vi "Taller 1 punto 4.vi"() -> ()   [LabVIEW 2017]
panel:
  out "Banda":dbl(slide) scale=0.0..1200.0
  in  "stop":bool
  in  "Velocidad (m/300ms)":dbl(knob) scale=0.0..10.0
  in  "Dirección":bool
  # "TALLER 1, PUNTO 4\nLUZ ANDREA JARAMILLO CASTILLO"
  # "Derecha"
  # "Izquierda"
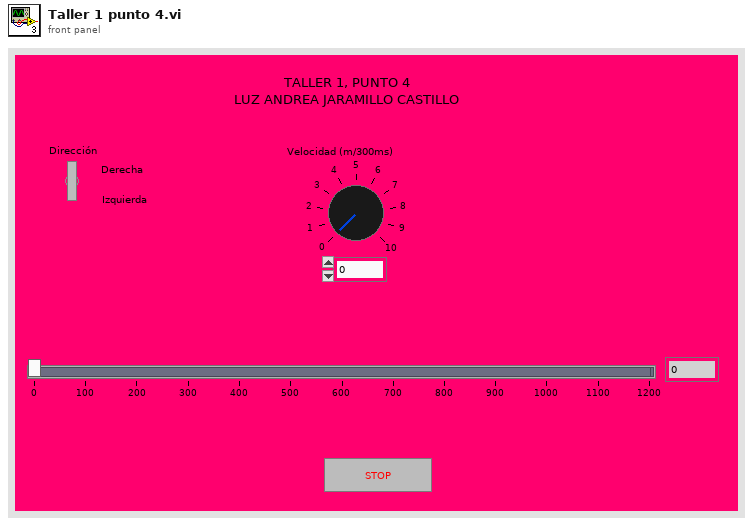
[diagram p1: front panel]
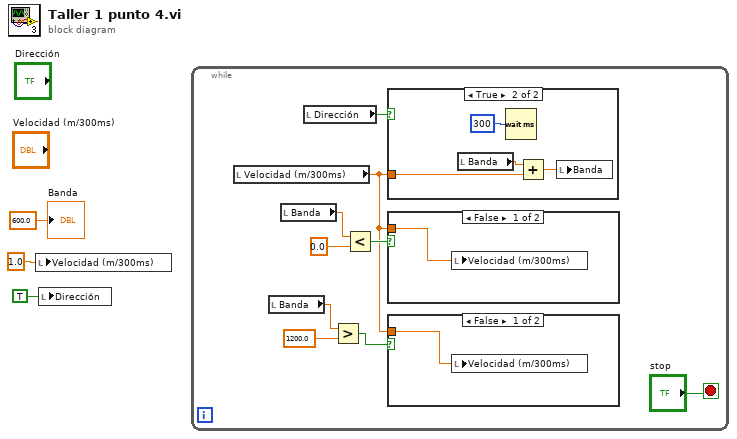
[diagram p0: block diagram]
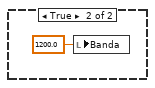
[diagram p2: hidden frame]
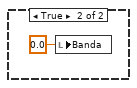
[diagram p3: hidden frame]
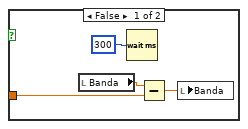
[diagram p4: hidden frame]
diagram:
  n1 = local write "Velocidad (m/300ms)"(1.0 ("Velocidad (m/300ms)")) -> ()
  n2 = local write "Dirección"(TRUE ("Dirección")) -> ()
  n3 = while {
    stop <- "stop" stop-if-true
    n4 = local read "Velocidad (m/300ms)"() -> (w4:dbl)
    n5 = local read "Banda"() -> (w8:dbl)
    n6 = local read "Banda"() -> (w9:dbl)
    n7 = local read "Dirección"() -> (w12:bool)
    n8 = Greater?(x=w8, y=1200.0) -> (0:w5:bool)
    n9 = Less?(x=w9, y=0.0) -> (x < y?=w6:bool)
    n10 = case shown="True" w12 {
      tunnel: w4 -> [w18 w21]
      frame False {
        n11 = local read "Banda"() -> (w17:dbl)
        n12 = Wait (ms)(milliseconds to wait=u32 300) -> ()  [unwired: 1 out]
        n13 = Subtract(x=w17, y=w18) -> (x-y=w20:dbl)
        n14 = local write "Banda"(w20) -> ()
      }
      frame True {
        n15 = local read "Banda"() -> (w24:dbl)
        n16 = Wait (ms)(milliseconds to wait=u32 300) -> ()  [unwired: 1 out]
        n17 = Add(x=w24, y=w21) -> (x+y=w23:dbl)
        n18 = local write "Banda"(w23) -> ()
      }
    }
    n19 = case shown="False" w6 {
      tunnel: w4 -> [w15 _]
      frame False {
        n20 = local write "Velocidad (m/300ms)"(w15) -> ()
      }
      frame True {
        n21 = local write "Banda"(0.0 ("Banda")) -> ()
      }
    }
    n22 = case shown="False" w5 {
      tunnel: w4 -> [w13 _]
      frame False {
        n23 = local write "Velocidad (m/300ms)"(w13) -> ()
      }
      frame True {
        n24 = local write "Banda"(1200.0 ("Banda")) -> ()
      }
    }
  }
  "Banda" <- 600.0 ("Slide")
